vi "4.2. CSM API String (Float with Unit) to Float.vi"() -> ()   [LabVIEW 2017]
doc: "### Float Type with Units in API String (4.2. CSM API String (Float with Unit) to Float.vi)\n\n#### Overview\n\nDemonstrates the conversion of floating-point numbers with units into floating-point numbers.\n\n#### Introduction\n\nCSM supports parsing floating-point numbers with units.\n\nIf there is a space between the floating-point string and the unit string, everything following the floating-point number (including symbols) is recognized as the unit string. For example:\n\n- `1.23mA` : Float: 1.23m; Unit: A\n- `1.23 mA` : Float: 1.23; Unit: mA\n\nFor floating-point numbers expressed in scientific notation, the string following the number is recognized as the unit string, regardless of whether a space exists. For example:\n\n- `1.23E+5mA`: Float: 1.23E+5; Unit: mA\n- `1.23E+5 mA`: Float: 1.23E+5; Unit: mA\n\nSpecial floating-point values such as `e`, `-e`, `pi`, `-pi`, `inf`, `+inf`, `-inf`, and `NaN` do not support units.\n\n#### Steps\n\n- step1: Testing floating-point unit conversion in various scenarios.\n- step2: The conversion in the API String depends on `String To Float_csm.vi`, available on the Functions palette."
uses:
  addons/API-String-Arugments-Support/API String Arguments Support.lvlib
panel:
  out "Example List":T1(array[cluster])=[{"CSM API String"="1.24A", "Float"=1.24, "Unit String"="A"}, {"CSM API String"="1.2KHz", "Float"=1200.0, "Unit String"="Hz"}, {"CSM API String"="1.2kHz", "Float"=1200.0, "Unit String"="Hz"}, {"CSM API String"="1.2 kHz", "Float"=1.2, "Unit String"="kHz"}, {"CSM API String"="243Ω", "Float"=243.0, "Unit String"="Ω"}, {"CSM API String"="12 mV", "Float"=12.0, "Unit String"="mV"}, {"CSM API String"="12mV", "Float"=0.012, "Unit String"="V"}, {"CSM API String"="1.23456435E+5A", "Float"=123456.43500000001, "Unit String"="A"}, {"CSM API String"="1.23456435E+5mA", "Float"=123456.43500000001, "Unit String"="mA"}, {"CSM API String"="1.23456435E+5 mA", "Float"=123456.43500000001, "Unit String"="mA"}]
  # "#CSM-Example Overview\n\nDemonstrates the conversion of floating-point numbers with units into floating-point numbers."
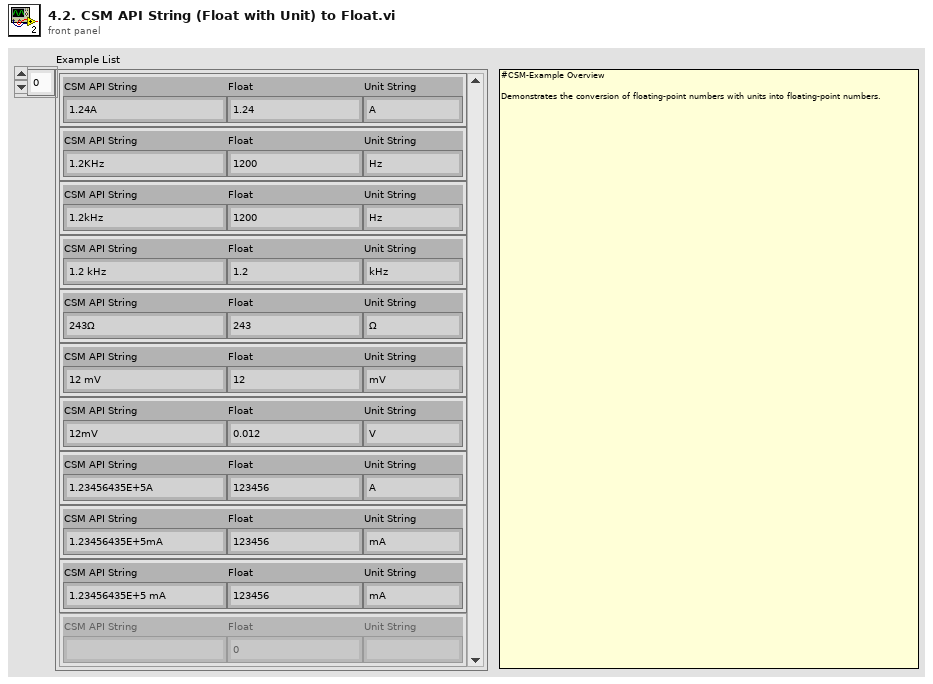
[diagram p1: front panel]
types:
  T1 = cluster{"CSM API String":string, "Float":dbl, "Unit String":string}[]
  T2 = cluster{"String":string, "Float":dbl, "Unit String":string}
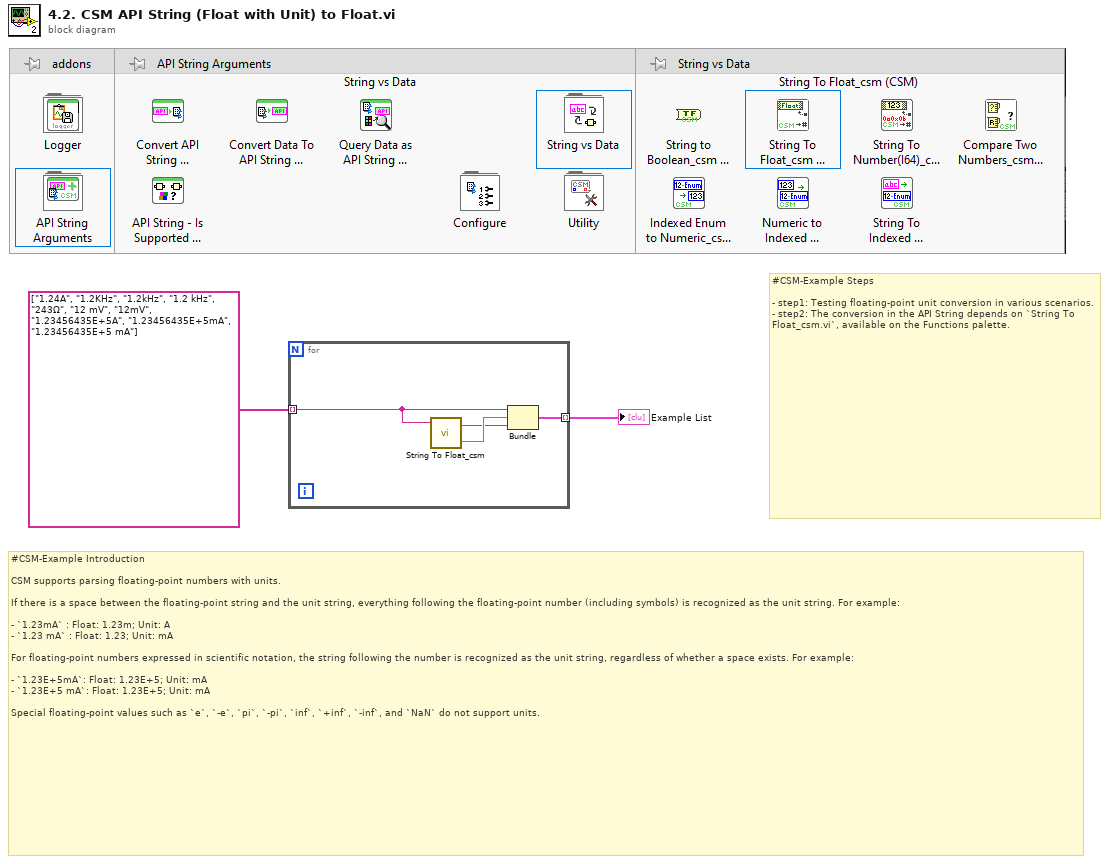
[diagram p0: block diagram]
diagram:
  # "#CSM-Example Steps\n\n- step1: Testing floating-point unit conversion in various scenarios.\n- step2: The conversion in the API String depends on `String To Float_csm.vi`, available on the Functions palette."
  # "#CSM-Example Introduction\n\nCSM supports parsing floating-point numbers with units.\n\nIf there is a space between the floating-point string and the unit string, everything following the floating-point number (including symbols) is recognized as the unit string. For example:\n\n- `1.23mA` : Float: 1.23m; Unit: A\n- `1.23 mA` : Float: 1.23; Unit: mA\n\nFor floating-point numbers expressed in scientific notation, the string following the number is recognized as the unit string, regardless of whether a space exists. For example:\n\n- `1.23E+5mA`: Float: 1.23E+5; Unit: mA\n- `1.23E+5 mA`: Float: 1.23E+5; Unit: mA\n\nSpecial floating-point values such as `e`, `-e`, `pi`, `-pi`, `inf`, `+inf`, `-inf`, and `NaN` do not support units."
  n1 = for {
    tunnel: string[] ["1.24A", "1.2KHz", "1.2kHz", "1.2 kHz", "243Ω", "12 mV", "12mV", "1.23456435E+5A", "1.23456435E+5mA", "1.23456435E+5 mA"] ("String") -> [w5] mode=indexing
    tunnel: [w6] -> w1 mode=indexing
    n2 = call "String To Float_csm.vi"("String"=w5) -> ("Float"=w4:dbl, "Unit String"=w3:string)  [unwired: 3 in]
    n3 = Bundle("String"=w5, "Float"=w4, "Unit String"=w3) -> (w6:T2)  [unwired: 1 in]
  }
  "Example List" <- w1
